vi "email errors.vi"(8 "error in (no error)":errorcluster, 11 "Loop id":string) -> (0 "error out (no error)":errorcluster)   [LabVIEW 2015]
uses:
  <vilib>/Utility/SMTP/NI_SMTPEmail.lvlib
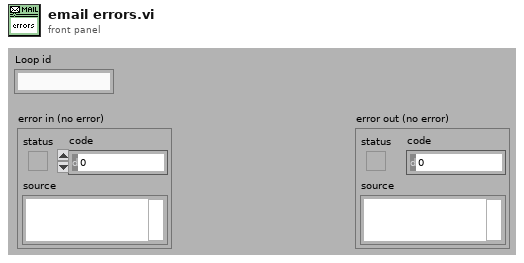
[diagram p1: front panel]
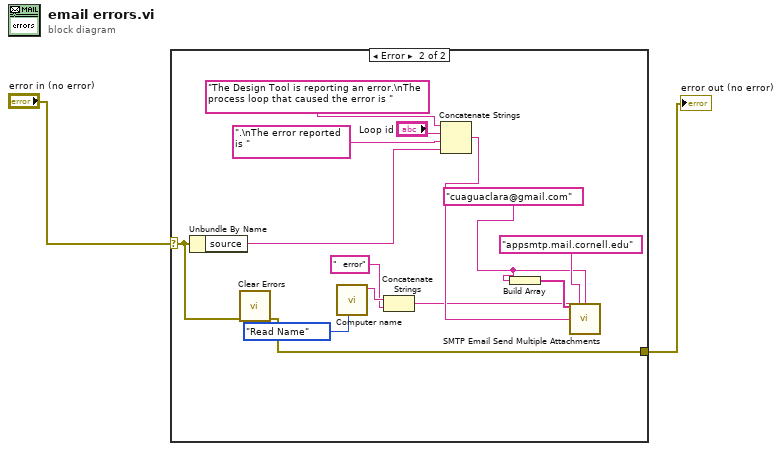
[diagram p0: block diagram]
diagram:
  n1 = case shown="Error" "error in (no error)" {
    selector: "error in (no error)" -> [w3 w9]
    tunnel: [w3 w8] -> w1
    frame No Error {
    }
    frame Error {
      w15 = "cuaguaclara@gmail.com" ("return address")
      n2 = Unbundle By Name(w9) -> ("source"=w11:string)
      n3 = call <vilib>:"Clear Errors.vi"("error in (no error)"=w9) -> ("error out"=w8:errorcluster)  [unwired: 5 in, 1 out]
      n4 = call "Computer name.vi"("cmd"=enum16{"Load Name", "Read Name"}."Read Name") -> ("Computer name"=w7:string)  [unwired: 9 in, 1 out]
      n5 = Concatenate Strings(w7, "  error" ("subject ([No Subject])")) -> (w5:string)
      n6 = Concatenate Strings("The Design Tool is reporting an error.\nThe process loop that caused the error is ", "Loop id", ".\nThe error reported is ", w11) -> (w10:string)
      n7 = Build Array(w15) -> (w17:string[])
      n8 = call <vilib>:"SMTP Email Send Multiple Attachments.vi"("recipients"=w17, "mail server"="appsmtp.mail.cornell.edu", "return address"=w15, "subject ([No Subject])"=w5, "message"=w10) -> ()  [unwired: 9 in, 2 out]
    }
  }
  "error out (no error)" <- w1
